vi "WristControl.vi"(4 "Pivot Angle":dbl, 5 "Disable Wrist Forward":bool, 6 "Wrist Angle (relative to ground)":dbl, 7 "Disable Wrist Back":bool, 8 "error in (no error)":errorcluster, 9 "Wrist Multiplier (degrees/second)":dbl=0.07, 10 "Wrist Stick":cluster{"X":dbl, "Y":dbl}, 11 "MotorControlDevRef":T1={"DeviceStatus"={"status"=FALSE, "code"=0, "source"=""}, "Type"=enum."PWM", "PWM"={"PWM Channel"=enum."Invalid", "DeadBand"={"Name"="", "maxPositivePwm"=0, "minPositivePwm"=0, "centerPwm"=0, "maxNegativePwm"=0, "minNegativePwm"=0, "angularRange"=0}}, "CAN"={"Device Number"=0, "Control Mode"=enum."Percent VBus", "Semaphore"=refnum, "Max Vout"=12.0, "TalonSRX Control Mode"=enum."Percent VBus"}, "Invert"=FALSE, "TransformRef"=refnum, "InvTransformRef"=refnum}) -> (0 "error out":errorcluster, 2 "Target Wrist Angle (relative to ground)":dbl, 3 "MotorControlDevRef":T1={"DeviceStatus"={"status"=FALSE, "code"=0, "source"=""}, "Type"=enum."PWM", "PWM"={"PWM Channel"=enum."Invalid", "DeadBand"={"Name"="", "maxPositivePwm"=0, "minPositivePwm"=0, "centerPwm"=0, "maxNegativePwm"=0, "minNegativePwm"=0, "angularRange"=0}}, "CAN"={"Device Number"=0, "Control Mode"=enum."Percent VBus", "Semaphore"=refnum, "Max Vout"=12.0, "TalonSRX Control Mode"=enum."Percent VBus"}, "Invert"=FALSE, "TransformRef"=refnum, "InvTransformRef"=refnum})   [LabVIEW 2015]
uses:
  <vilib>/Rock Robotics/WPI/MotorControl/WPI_MotorControlDeviceRef.ctl
  <vilib>/Rock Robotics/WPI/MotorControl/WPI_MotorControlType.ctl
  <vilib>/Rock Robotics/SystemInterfaces/DIO/FPGA_DIOPWMChannel.ctl
  <vilib>/Rock Robotics/WPI/PWM/WPI_PWMDeadband.ctl
  <vilib>/Rock Robotics/WPI/CAN/Jaguar/SubVIs/WPI_CANJaguar_ControlMode.ctl
  <vilib>/Rock Robotics/WPI/CAN/TalonSRX/WPI_CANTalonSRX_APIControlMode.ctl
  <vilib>/Rock Robotics/WPI/PWM/WPI_PWMTransform_ConPane.ctl
  Robot Global Data.vi
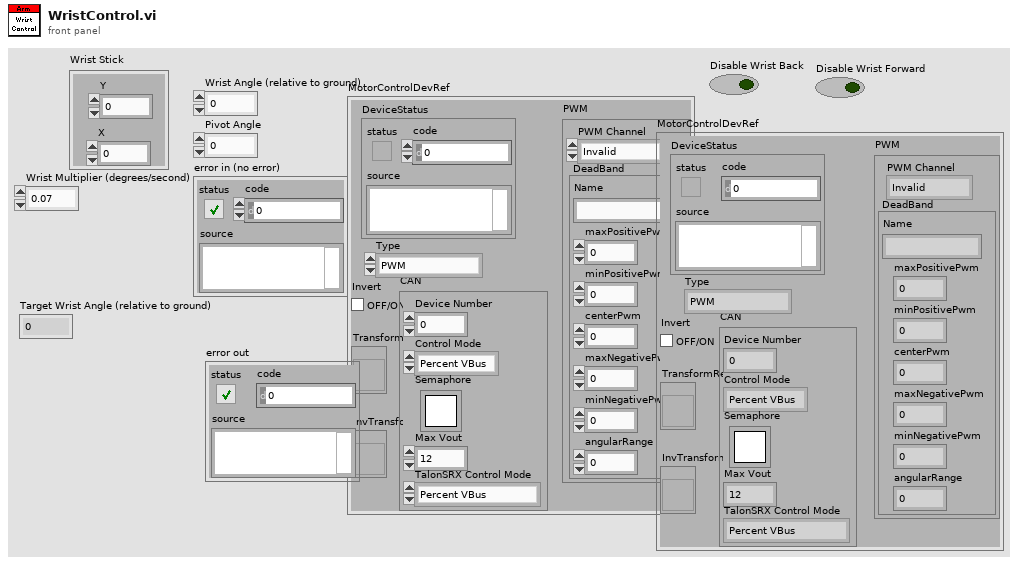
[diagram p1: front panel]
types:
  T1 = typedef "WPI_MotorControlDeviceRef.ctl" = cluster{"DeviceStatus":errorcluster, "Type":T2, "PWM":cluster{"PWM Channel":T3, "DeadBand":T4}, "CAN":cluster{"Device Number":u8, "Control Mode":T5, "Semaphore":T6, "Max Vout":dbl, "TalonSRX Control Mode":T7}, "Invert":bool, "TransformRef":T8, "InvTransformRef":T8}
  T2 = typedef "WPI_MotorControlType.ctl" = enum16{"PWM", "CAN", "CANTalonSRX"}
  T3 = typedef "FPGA_DIOPWMChannel.ctl" = enum8{"PWM 0", "PWM 1", "PWM 2", "PWM 3", "PWM 4", "PWM 5", "PWM 6", "PWM 7", "PWM 8", "PWM 9", "PWM MXP 0", "PWM MXP 1", "PWM MXP 2", "PWM MXP 3", "PWM MXP 4", "PWM MXP 5", "PWM MXP 6", "PWM MXP 7", "PWM MXP 8", "PWM MXP 9", "Invalid"}
  T4 = typedef "WPI_PWMDeadband.ctl" = cluster{"Name":string, "maxPositivePwm":i32, "minPositivePwm":i32, "centerPwm":i32, "maxNegativePwm":i32, "minNegativePwm":i32, "angularRange":u16}
  T5 = typedef "WPI_CANJaguar_ControlMode.ctl" = enum8{"Percent VBus", "Current", "Speed", "Position", "Voltage"}
  T6 = typedef "Semaphore RefNum" = refnum<k1>
  T7 = typedef "WPI_CANTalonSRX_APIControlMode.ctl" = enum8{"Percent VBus", "Speed", "Position", "Slave", "Unchanged / Invalid"}
  T8 = typedef "WPI_PWMTransform_ConPane.ctl" = refnum<vi>
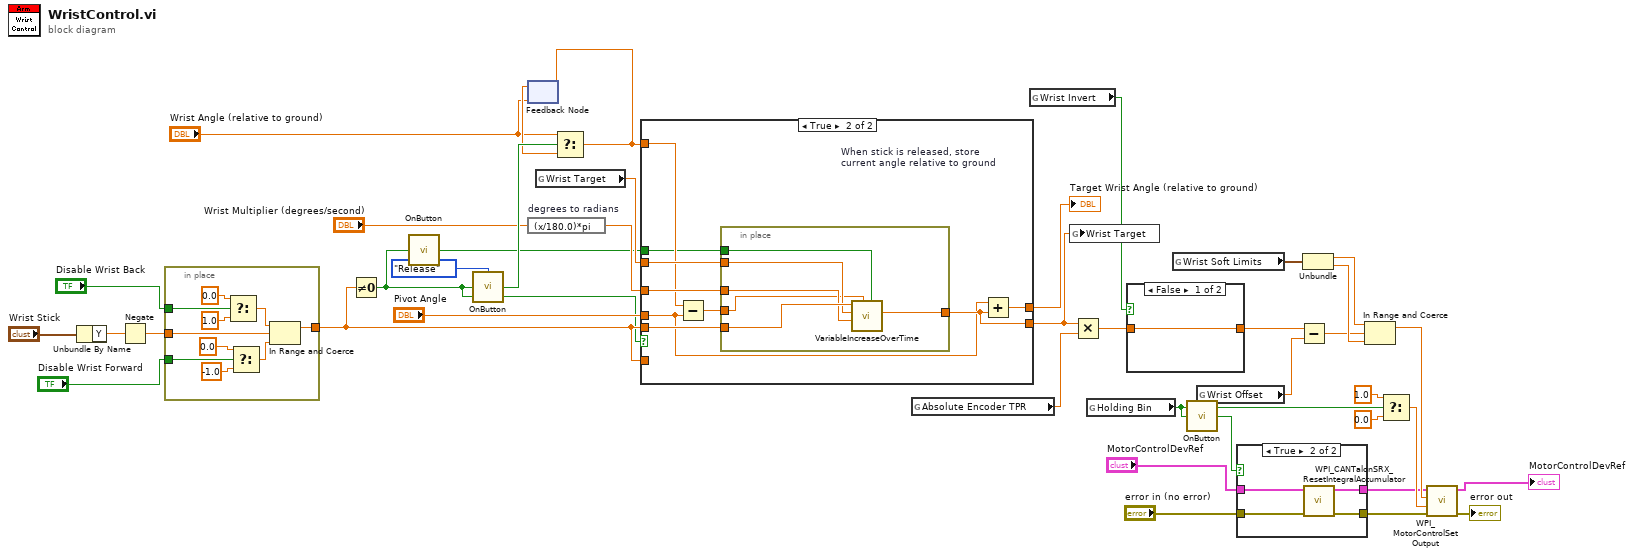
[diagram p0: block diagram]
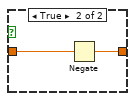
[diagram p2: hidden frame]
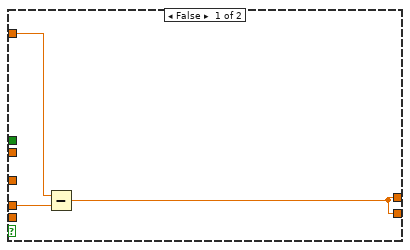
[diagram p4: hidden frame]
diagram:
  n1 = Unbundle By Name("Wrist Stick") -> ("Y"=w40:dbl)
  n2 = Negate(x=w40) -> (-x=w33:dbl)
  n3 = in-place {
    in-place-border: [w48] -> w16
    in-place-border: w33 -> [w47]
    in-place-border: "Disable Wrist Forward" -> [w42]
    in-place-border: "Disable Wrist Back" -> [w41]
    n4 = Select(t=0.0, s=w41, f=1.0) -> (s? t:f=w50:dbl)
    n5 = Select(t=0.0, s=w42, f=-1.0) -> (s? t:f=w49:dbl)
    n6 = In Range and Coerce(upper limit=w50, x=w47, lower limit=w49) -> (coerced(x)=w48:dbl)  [unwired: 1 out]
  }
  n7 = Not Equal To 0?(x=w16) -> (x != 0?=w8:bool)
  n8 = call "OnButton.vi"("Button"=w8) -> ("Value"=w7:bool)  [unwired: 1 in]
  n9 = call "OnButton.vi"("Button"=w8, "Mode"=enum16{"Press", "Release", "Both"}."Release") -> ("Value"=w32:bool)
  n10 = feedback #1 "When stick is released, store \ncurrent angle relative to ground"("Wrist Angle (relative to ground)") -> (w31:dbl)
  n11 = expression code="(x/180.0)*pi" "degrees to radians"("Wrist Multiplier (degrees/second)") -> (w15:dbl)
  n12 = global read "Robot Global Data.vi" "Wrist Target"() -> (w18:dbl)
  n13 = Select(t="Wrist Angle (relative to ground)", s=w32, f=w31) -> (s? t:f=w6:dbl)
  n14 = feedback-in #1(w6) -> ()
  n15 = case shown="True" w8 {
    tunnel: [w51 w59] -> w23
    tunnel: w6 -> [w53 w57]
    tunnel: w16 -> [_ _]
    tunnel: "Pivot Angle" -> [w52 w56]
    tunnel: [w51 w58] -> w4
    tunnel: w18 -> [_ w61]
    tunnel: w16 -> [_ w62]
    tunnel: w15 -> [_ w60]
    tunnel: w7 -> [_ w54]
    frame False {
      n16 = Subtract(x=w53, y=w52) -> (x-y=w51:dbl)
    }
    frame True {
      n17 = Subtract(x=w57, y=w56) -> (x-y=w55:dbl)
      n18 = in-place {
        in-place-border: w62 -> [w67]
        in-place-border: [w68] -> w58
        in-place-border: w61 -> [w66]
        in-place-border: w60 -> [w65]
        in-place-border: w55 -> [w64]
        in-place-border: w54 -> [w63]
        n19 = call "VariableIncreaseOverTime.vi"("Reset to current"=w63, "Current value"=w64, "Multiplier (units/sec)"=w65, "Variable in"=w66, "Joystick input"=w67) -> ("Variable out"=w68:dbl)  [unwired: 6 in]
      }
      n20 = Add(x=w56, y=w58) -> (x+y=w59:dbl)
    }
  }
  "Target Wrist Angle (relative to ground)" <- w23
  n21 = global read "Robot Global Data.vi" "Absolute Encoder TPR"() -> (w26:dbl)
  n22 = global read "Robot Global Data.vi" "Wrist Invert"() -> (w1:bool)
  n23 = global write "Robot Global Data.vi" "Wrist Target"(w4) -> ()
  n24 = Multiply(x=w4, y=w26) -> (x*y=w3:dbl)
  n25 = global read "Robot Global Data.vi" "Holding Bin"() -> (w14:bool)
  n26 = case shown="False" w1 {
    tunnel: w3 -> [w69 w71]
    tunnel: [w69 w70] -> w2
    frame False {
    }
    frame True {
      n27 = Negate(x=w71) -> (-x=w70:dbl)
    }
  }
  n28 = global read "Robot Global Data.vi" "Wrist Soft Limits"() -> (w30:cluster{"Forward":dbl, "Reverse":dbl})
  n29 = call "OnButton.vi"("Button"=w14) -> ("Value"=w13:bool)  [unwired: 1 in]
  n30 = global read "Robot Global Data.vi" "Wrist Offset"() -> (w25:dbl)
  n31 = case shown="True" w13 {
    tunnel: "error in (no error)" -> [w73 w77]
    tunnel: [w73 w76] -> w11
    tunnel: "MotorControlDevRef" -> [w72 w75]
    tunnel: [w72 w74] -> w9
    frame False {
    }
    frame True {
      n32 = call <vilib>:"WPI_CANTalonSRX_ResetIntegralAccumulator.vi"("error in (no error)"=w77, "CAN Talon SRX Ref"=w75) -> ("error out"=w76:errorcluster, "CAN Talon SRX Ref"=w74:T1)  [unwired: 8 in]
    }
  }
  n33 = Subtract(x=w2, y=w25) -> (x-y=w24:dbl)
  n34 = Unbundle(w30) -> ("Forward"=w28:dbl, "Reverse"=w29:dbl)
  n35 = In Range and Coerce(upper limit=w28, x=w24, lower limit=w29) -> (coerced(x)=w27:dbl)  [unwired: 1 out]
  n36 = Select(t=1.0, s=w14, f=0.0) -> (s? t:f=w20:dbl)
  n37 = call <vilib>:"WPI_MotorControlSetOutput.vi"("error in (no error)"=w11, "Sync Group / Parameter Slot"=w20, "Output"=w27, "MotorControlDevRef"=w9) -> ("error out"=→"error out":errorcluster, "MotorControlDevRef"=→"MotorControlDevRef":T1)  [unwired: 5 in, 1 out]
